vi "ThrustReadout.vi"(4 "LabJack Supply":dbl, 5 "k":dbl, 6 "error in":errorcluster, 7 "AIN Range":u16(ring) items=["LJ_rgBIP10V", "LJ_rgBIP1V", "LJ_rgBIPP1V", "LJ_rgBIPP01V"], 8 "+Channel":u16, 9 "Handle In":i32) -> (0 "error out":errorcluster, 1 "Voltage Reading":dbl, 2 "Displacement Reading [meter]":dbl, 3 "Thrust Reading [Newton]":dbl)   [LabVIEW 2021]
panel:
  # "inputs"
  # "outputs"
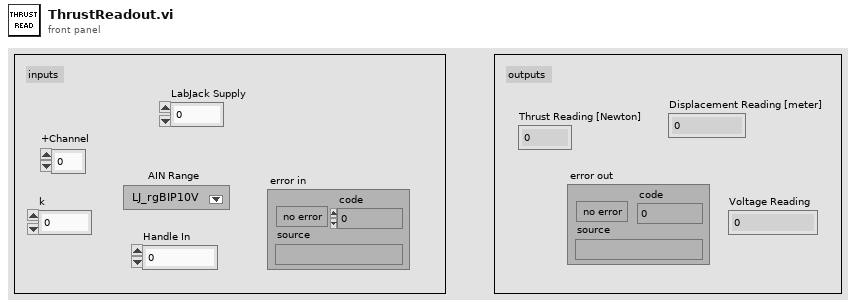
[diagram p1: front panel]
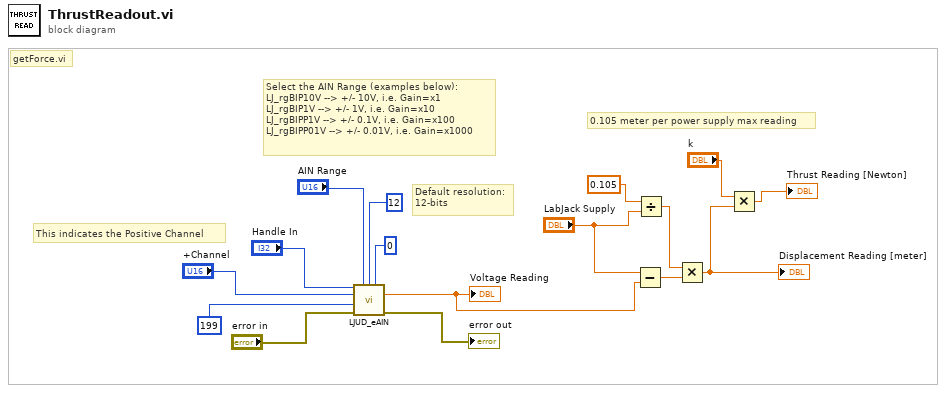
[diagram p0: block diagram]
diagram:
  # "0.105 meter per power supply max reading"
  # "getForce.vi"
  # "This indicates the Positive Channel"
  # "Default resolution:\n12-bits"
  # "Select the AIN Range (examples below):\nLJ_rgBIP10V --> +/- 10V, i.e. Gain=x1\nLJ_rgBIP1V --> +/- 1V, i.e. Gain=x10\nLJ_rgBIPP1V --> +/- 0.1V, i.e. Gain=x100\nLJ_rgBIPP01V --> +/- 0.01V, i.e. Gain=x1000"
  n1 = call <vilib>:"LJUD_eAIN.vi"("Handle In"="Handle In", "Range"="AIN Range", "Resolution"=12, "Settling"=0, "ChannelP"="+Channel", "ChannelN"=199, "error in"="error in") -> ("Voltage"=w2:dbl, "error out"=→"error out":errorcluster)  [unwired: 6 in, 1 out]
  "Voltage Reading" <- w2
  n2 = Subtract(x="LabJack Supply", y=w2) -> (x-y=w3:dbl)
  n3 = Divide(x=0.105, y="LabJack Supply") -> (x/y=w7:dbl)
  n4 = Multiply(x=w7, y=w3) -> (x*y=w5:dbl)
  "Displacement Reading [meter]" <- w5
  n5 = Multiply(x="k", y=w5) -> (x*y=→"Thrust Reading [Newton]":dbl)
